vi "Create Fake Instrument.vi"(8 "error in":errorcluster, 10 "provided interface":string="fake_interface", 11 "instrument type id":string="fake_instrument_type") -> (0 "error out":errorcluster, 3 "fake instrument out":refnum<class "Fake Instrument.lvclass">)   [LabVIEW 2020, in "MeasurementServerTests.lvlib" / "Fake Instrument.lvclass"]
uses:
  Fake Instrument.lvclass
  Fake Instrument.lvclass/Fake Instrument.ctl
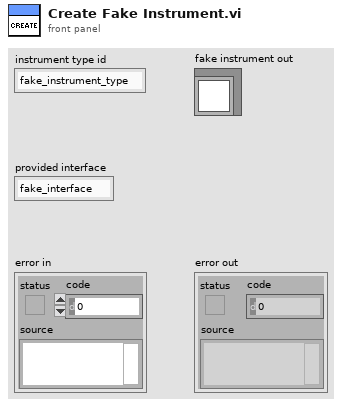
[diagram p1: front panel]
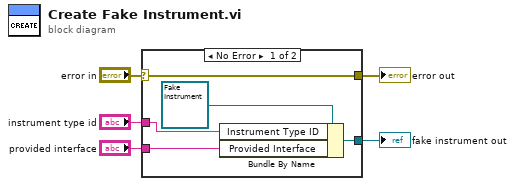
[diagram p0: block diagram]
diagram:
  n1 = case shown="No Error" "error in" {
    selector: "error in" -> [w10 w11]
    tunnel: [w10 w11] -> w4
    tunnel: [w8 _] -> w3
    tunnel: "instrument type id" -> [w7 _]
    tunnel: "provided interface" -> [w6 _]
    frame No Error {
      n2 = Bundle By Name(cluster=refnum<class "Fake Instrument.lvclass"> refnum ("fake instrument out"), "Instrument Type ID"=w7, "Provided Interface"=w6) -> (w8:refnum<class "Fake Instrument.lvclass">)
    }
    frame Error {
    }
  }
  "error out" <- w4
  "fake instrument out" <- w3
